vi "4.2.2.vi"() -> ()   [LabVIEW 2017]
panel:
  in  "Phase 2":dbl
  in  "Phase 1":dbl
  out "XY Graph":cluster{"X":dbl[], "Y":dbl[]}[](graph)
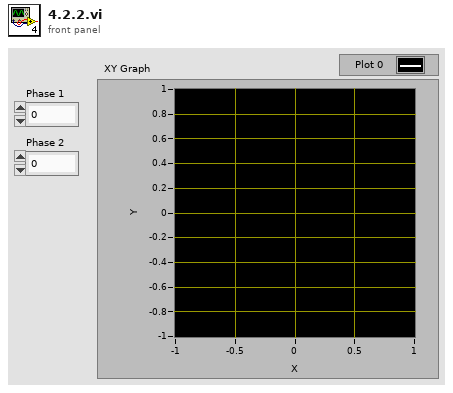
[diagram p1: front panel]
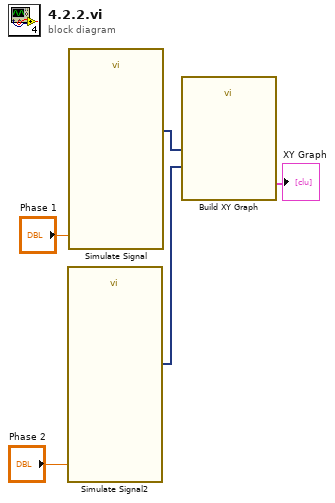
[diagram p0: block diagram]
diagram:
  n1 = call "Simulate Signal2"("Phase"="Phase 2") -> ("Sine"=w4:dynamicdata)  [unwired: 13 in, 1 out]
  n2 = call "Simulate Signal"("Phase"="Phase 1") -> ("Sine"=w5:dynamicdata)  [unwired: 13 in, 1 out]
  n3 = call "Build XY Graph"("Y Input"=w4, "X Input"=w5) -> ("XY Graph"=→"XY Graph":cluster{"X":dbl[], "Y":dbl[]}[])  [unwired: 8 in, 1 out]
